vi "Flash Start Stream.vi"(8 "error in (no error)":errorcluster, 9 "File Path":path, 10 "Camera Settings":T1={"Exposure Time (ms)"=100.0, "Binning"=enum."2x2", "Scan Mode"=0, "Frames to Acquire"=1000.0, "Pixel Correction"=FALSE, "Frames to Skip"=0, "File Path"=path "", "Duty cycle"=0.0, "ALEX"=FALSE, "Shutter Enable"=[]} {"Exposure Time (ms)" min=1.0 max=10000.0 step=1.0}, 11 "Orca-Flash 4.0 V2 in":refnum<class "Orca-Flash 4.0 V2.lvclass">) -> (0 "error out":errorcluster, 3 "Orca-Flash 4.0 V2 out":refnum<class "Orca-Flash 4.0 V2.lvclass">)   [LabVIEW 2018, in "Orca-Flash 4.0 V2.lvlib" / "Orca-Flash 4.0 V2.lvclass"]
uses:
  Orca-Flash 4.0 V2.lvclass
  C:/LVCUR/flash-gordon/Hardware/Camera/Camera.lvclass
  Resources/Type Defs/Camera Settings.ctl
  Orca-Flash 4.0 V2.lvclass/Orca-Flash 4.0 V2.ctl
  Resources/GLOBAL/GLOBAL Time-critical.vi
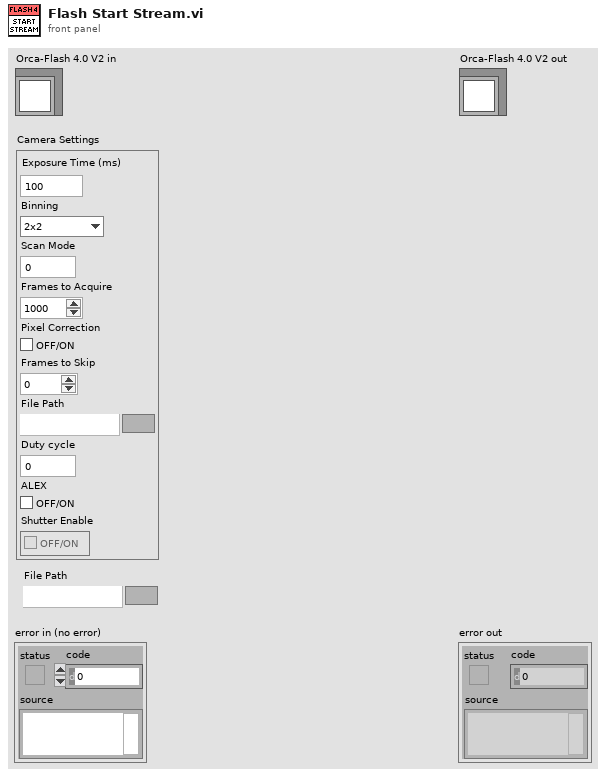
[diagram p1: front panel]
types:
  T1 = typedef "Camera Settings.ctl" = cluster{"Exposure Time (ms)":dbl, "Binning":enum16{"1x1", "2x2", "4x4"}, "Scan Mode":i32, "Frames to Acquire":dbl, "Pixel Correction":bool, "Frames to Skip":u32, "File Path":path, "Duty cycle":dbl, "ALEX":bool, "Shutter Enable":bool[]}
  T2 = typedef "Physical Camera Assignment.ctl" = cluster{"Channel Name":string, "Camera Type":T3, "Serial Number":string, "Flip Vertically":bool, "Flip Horizontally":bool, "photonsPerCount":dbl, "wavelength":i16}
  T3 = typedef "Camera Type.ctl" = enum16{"Orca-Flash 4.0 V2"}
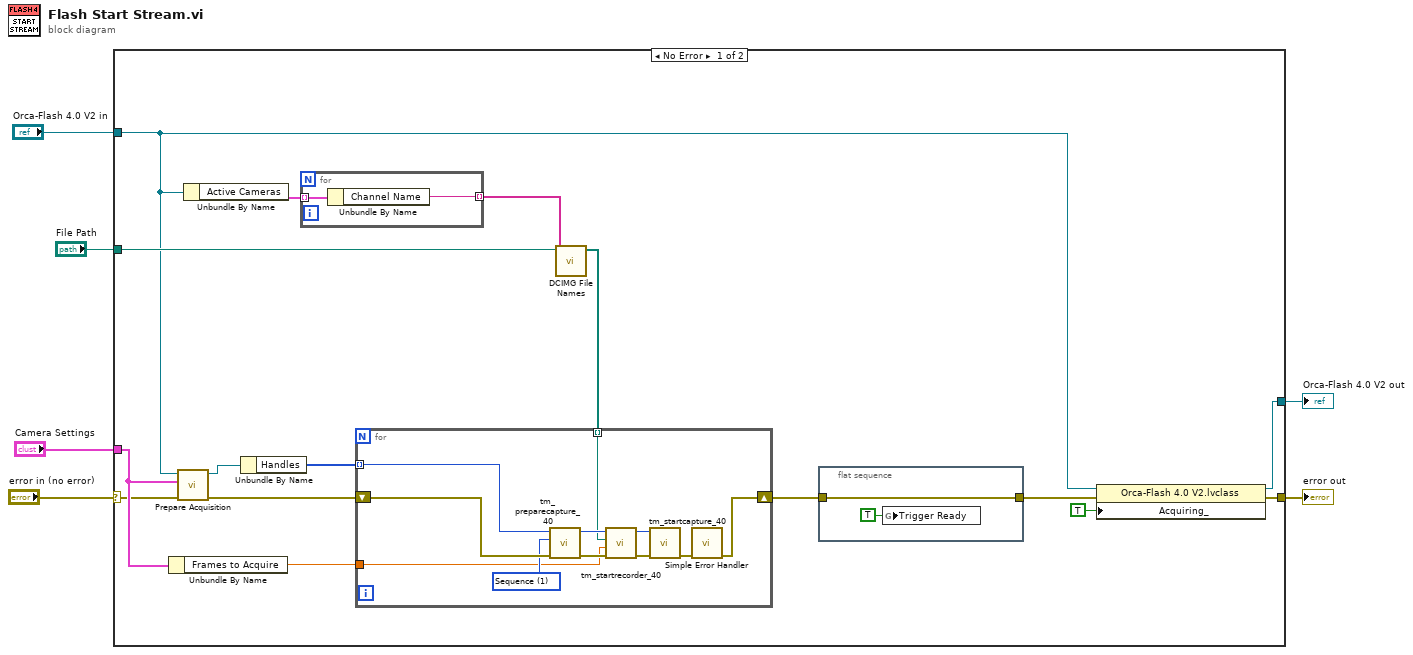
[diagram p0: block diagram]
diagram:
  n1 = case shown="No Error" "error in (no error)" {
    selector: "error in (no error)" -> [w19 w39]
    tunnel: [w18 w39] -> w5
    tunnel: [w17 w38] -> w3
    tunnel: "Orca-Flash 4.0 V2 in" -> [w8 w38]
    tunnel: "File Path" -> [w13 _]
    tunnel: "Camera Settings" -> [w20 _]
    frame No Error {
      n2 = Unbundle By Name(w20) -> ("Frames to Acquire"=w14:dbl)
      n3 = call "Prepare Acquisition.vi"("error in (no error)"=w19, "Flash Settings"=w20, "Orca-Flash 4.0 in"=w8) -> ("error out"=w16:errorcluster, "Orca-Flash 4.0 out"=w22:refnum<class "Orca-Flash 4.0 V2.lvclass">)  [unwired: 7 in]
      n4 = Unbundle By Name(w8) -> ("Active Cameras"=w7:T2[])
      n5 = Unbundle By Name(w22) -> ("Handles"=w15:u32[])
      n6 = for {
        tunnel: [w37] -> w11 mode=indexing
        tunnel: w7 -> [w36] mode=indexing
        n7 = Unbundle By Name(w36) -> ("Channel Name"=w37:string)
      }
      n8 = call "DCIMG File Names.vi"("Channel Names"=w11, "TIFF File Path"=w13) -> ("DCIMG Files"=w12:path[])  [unwired: 9 in]
      n9 = for {
        tunnel: w15 -> [w30] mode=indexing
        tunnel: w14 -> [w27]
        shift-right: [w26] -> w10
        shift-left: w16 -> [w35]
        tunnel: w12 -> [w25] mode=indexing
        w29 = 1 items=["Snap", "Sequence"] ("Capture mode")
        n10 = call <userlib>:"tm_preparecapture_40.vi"("error in (no error)"=w35, "Capture mode"=w29, "Handle in"=w30) -> ("error out"=w34:errorcluster, "Handle out"=w31:u32)  [unwired: 5 in, 2 out]
        n11 = call <userlib>:"tm_startrecorder_40.vi"("error in (no error)"=w34, "frames"=w27, "File"=w25, "Handle in"=w31) -> ("error out"=w33:errorcluster, "Handle out"=w32:u32)  [unwired: 6 in]
        n12 = call <userlib>:"tm_startcapture_40.vi"("error in (no error)"=w33, "Handle in"=w32) -> ("error out"=w28:errorcluster)  [unwired: 8 in, 1 out]
        n13 = call <vilib>:"Simple Error Handler.vi"("error in (no error)"=w28) -> ("error out"=w26:errorcluster)  [unwired: 4 in, 4 out]
      }
      n14 = flat-sequence {
        tunnel: w10 -> [w24]
        tunnel: [w24] -> w9
        frame #0 {
          n15 = global write "GLOBAL Time-critical.vi" "Trigger Ready"(TRUE ("new element/subarray")) -> ()
        }
      }
      n16 = property class="Orca-Flash 4.0 V2.lvclass"(reference=w8, error in=w9, "Acquiring_"=TRUE ("Live Mode")) -> (reference out=w17:refnum<class "Orca-Flash 4.0 V2.lvclass">, error out=w18:errorcluster)
    }
    frame Error {
    }
  }
  "error out" <- w5
  "Orca-Flash 4.0 V2 out" <- w3
